vi "Main.vi"(8 "error in":errorcluster, 11 "Main UI in":refnum<class "Main UI.lvclass">) -> (0 "error out":errorcluster, 3 "Main UI out":refnum<class "Main UI.lvclass">)   [LabVIEW 2019, in "Main UI.lvclass"]
doc: "The <b>Queued Message Handler</b> of the Worker that owns this VI."
uses:
  Main UI.lvclass
  C:/Program Files (x86)/National Instruments/LabVIEW 2019/vi.lib/addons/_Workers/Library/Classes/Worker/Worker.lvclass
  Initialization Data.ctl
  Response Cases.ctl
  <vilib>/addons/_Workers/Library/Case Label.ctl
  Main UI.lvclass/Main UI.ctl
  rql_Start Motor.ctl
  <vilib>/addons/_Workers/Library/Classes/Message Queue/Message Queue.lvclass
  <vilib>/addons/_Workers/Library/Workers.lvlib
panel:
  in  "Start Motor":bool
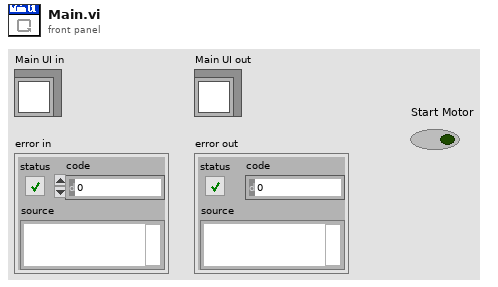
[diagram p1: front panel]
types:
  T1 = typedef "Main UI.lvclass/Initialization Data.ctl" = cluster{"Response Cases":T2}
  T2 = typedef "Main UI.lvclass/Response Cases.ctl" = cluster{"Placeholder - Can be deleted":string, "Start Motor":T3}
  T3 = typedef "Workers.lvlib/Case Label.ctl" = string
  T4 = typedef "Main UI.lvclass/rql_Start Motor.ctl" = cluster{"String":string}
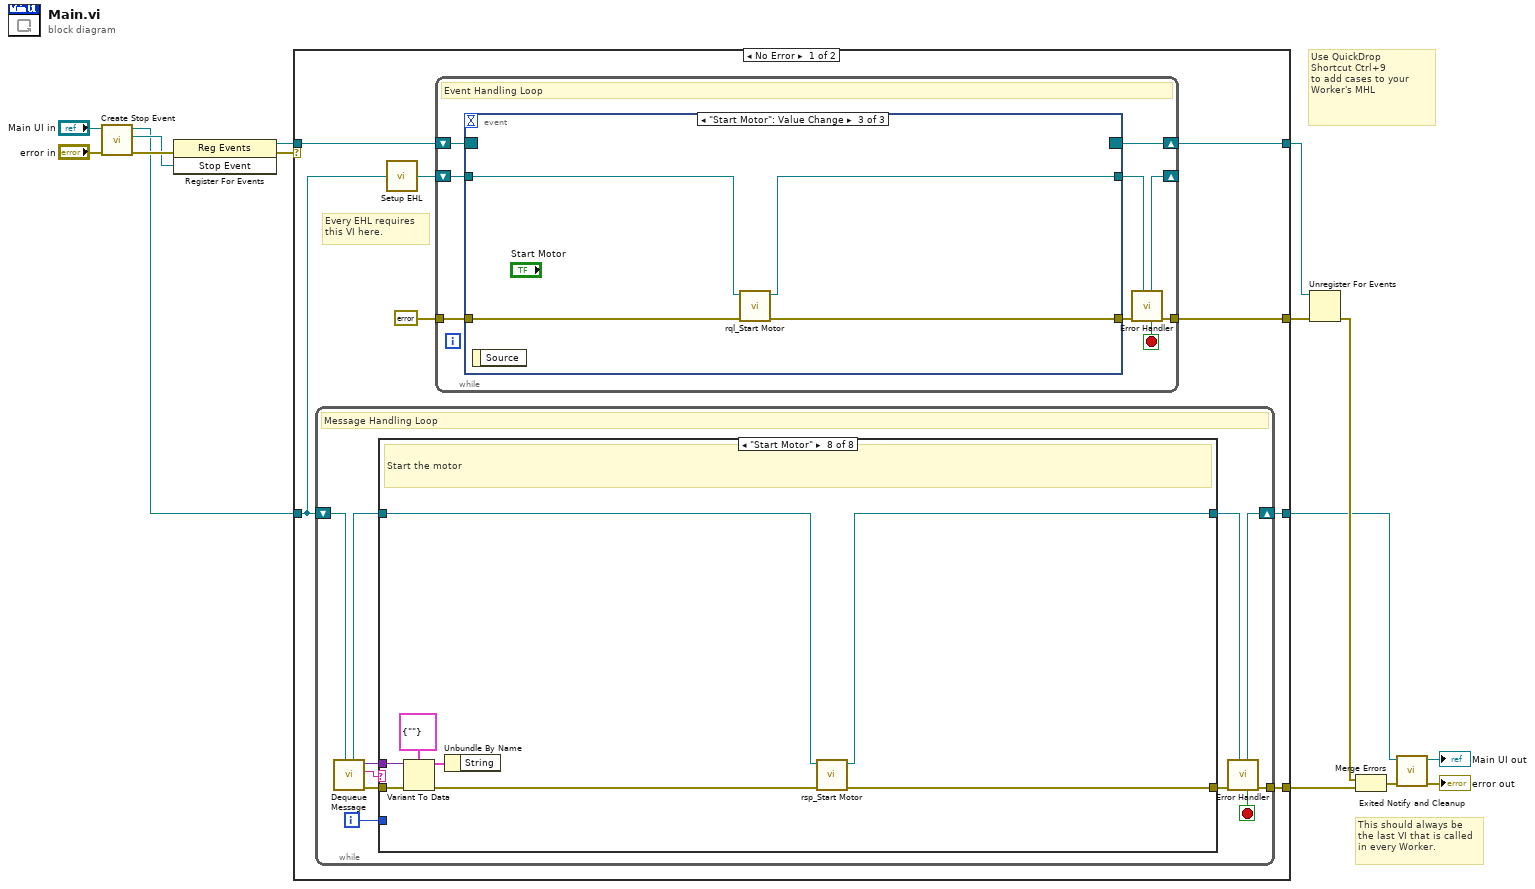
[diagram p0: block diagram]
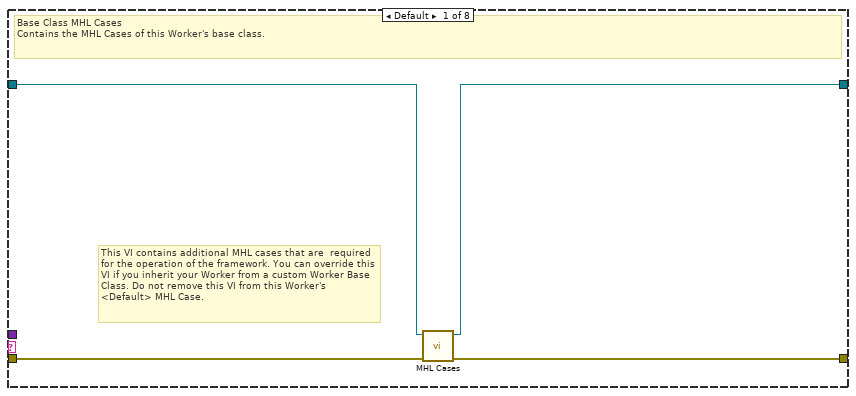
[diagram p2: hidden frame]
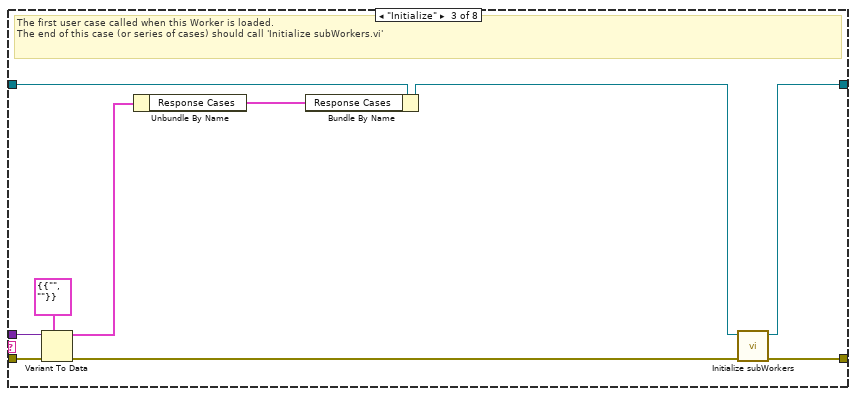
[diagram p4: hidden frame]
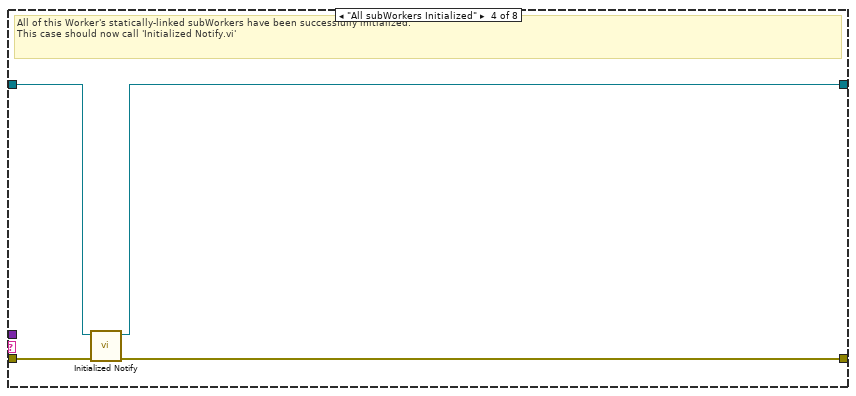
[diagram p5: hidden frame]
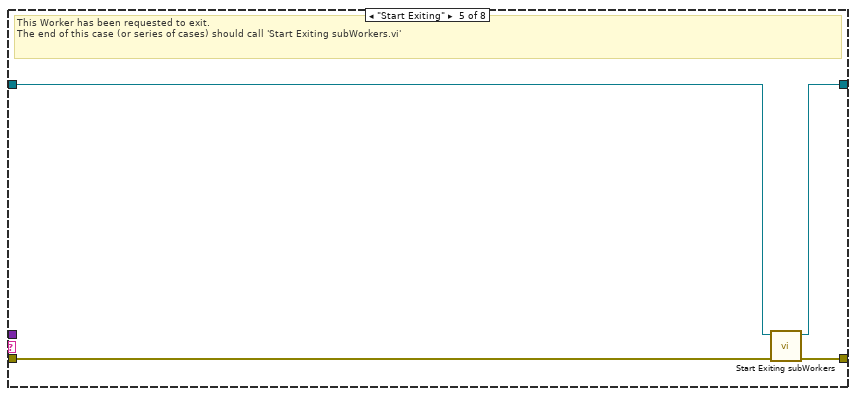
[diagram p6: hidden frame]
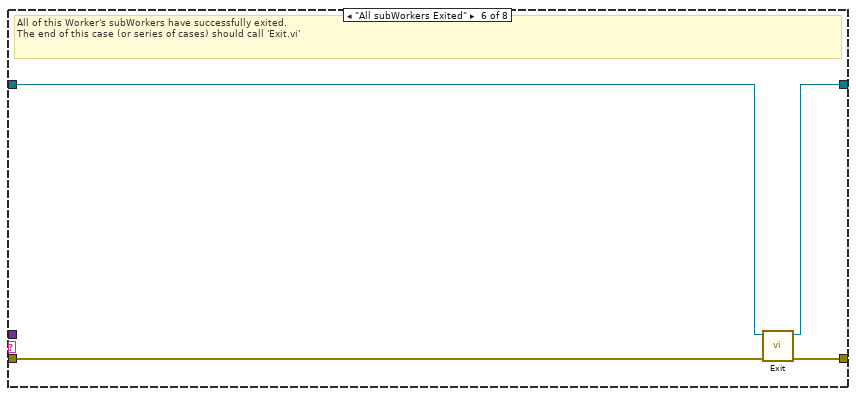
[diagram p7: hidden frame]
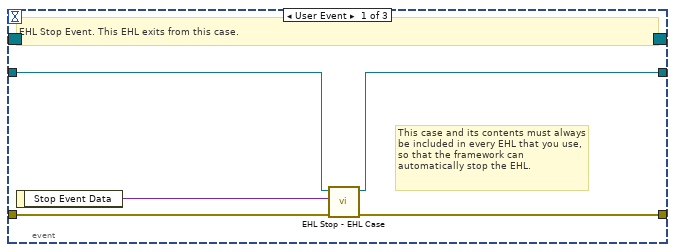
[diagram p9: hidden frame]
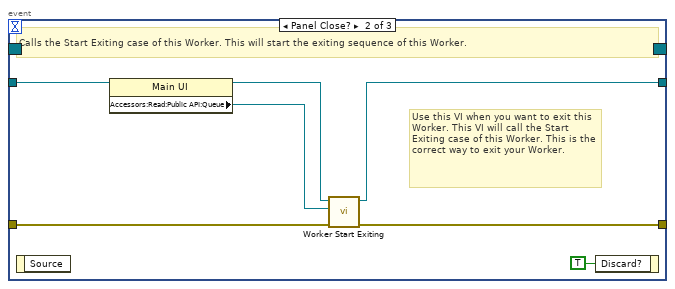
[diagram p10: hidden frame]
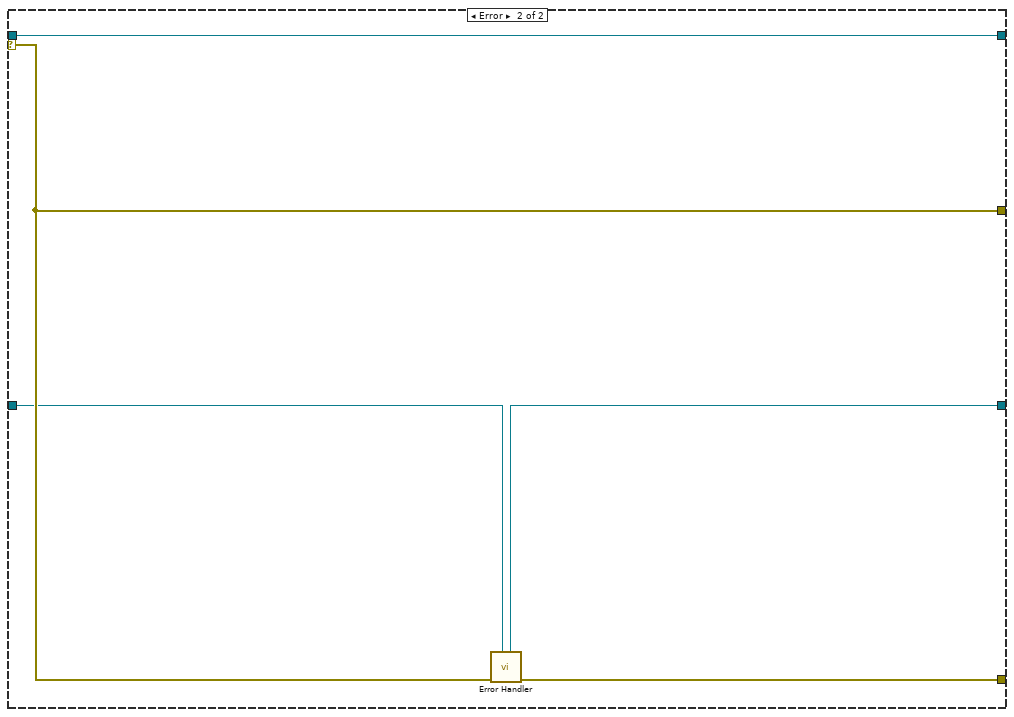
[diagram p11: hidden frame]
diagram:
  # "Use QuickDrop\nShortcut Ctrl+9\nto add cases to your\nWorker's MHL"
  # "This should always be the last VI that is called in every Worker."
  n1 = call-dynamic "Create Stop Event.vi"("error in"="error in", "Worker"="Main UI in") -> ("error out"=w10:errorcluster, "Stop Event"=w7:refnum<user-event>, "Worker out"=w4:refnum<class "Main UI.lvclass">)  [unwired: 7 in]
  n2 = register-events(error in=w10, w7) -> (reference out=w9:refnum<event-registration>, error out=w1:errorcluster)  [unwired: 1 in]
  n3 = case shown="No Error" w1 {
    tunnel: w4 -> [w18 w99]
    tunnel: [w16 w100] -> w8
    tunnel: w9 -> [w23 w101]
    tunnel: [w20 w102] -> w14
    tunnel: [w22 w101] -> w13
    tunnel: [w17 w98] -> w11
    selector: w1 -> [_ w102]
    frame No Error {
      # "Every EHL requires\nthis VI here."
      n4 = while {
        shift-right: [w32] -> w17
        shift-left: w18 -> [w34]
        tunnel: [w33] -> w16
        i -> [w25]
        stop <- w26 stop-if-true
        # "Message Handling Loop"
        n5 = call-dynamic "Dequeue Message.vi"("Worker"=w34) -> ("error out"=w31:errorcluster, "Case out"=w27:string, "Data out"=w24:variant, "Worker out"=w29:refnum<class "Main UI.lvclass">)  [unwired: 6 in, 1 out]
        n6 = case "Worker MHL Case Structure (DO NOT CHANGE LABEL NAME)" shown="\"Start Motor\"" w27 {
          tunnel: w31 -> [w38 w39 w48 w52 w55 w62 w64 w72]
          tunnel: [w37 w39 w50 w51 w58 w61 w64 w67] -> w30
          tunnel: w29 -> [w36 w40 w47 w54 w56 w60 w63 w66]
          tunnel: [w35 w40 w49 w53 w57 w59 w63 w65] -> w28
          tunnel: w25 -> [_ _ _ _ _ _ _ _]
          tunnel: w24 -> [_ _ w45 _ _ _ _ w70]
          frame Default {
            # "This VI contains additional MHL cases that are  required for the operation of the framework. You can override this VI if you inherit your Worker from a custom Worker Base Class. Do not remove this VI from this Worker's <Default> MHL Case."
            # "Base Class MHL Cases\nContains the MHL Cases of this Worker's base class."
            n7 = call-dynamic "MHL Cases.vi"("error in"=w38, "Worker in"=w36) -> ("error out"=w37:errorcluster, "Worker out"=w35:refnum<class "Main UI.lvclass">)  [unwired: 8 in]
          }
          frame "------------ FRAMEWORK CASES -----------" {
            # "Start of Workers Framework Cases"
          }
          frame "Initialize" {
            # "The first user case called when this Worker is loaded.\nThe end of this case (or series of cases) should call 'Initialize subWorkers.vi'"
            n8 = Variant To Data(error in=w48, type=T1 {"Response Cases"={"Placeholder - Can be deleted"="", "Start Motor"=""}} ("Initialization Data"), Variant=w45) -> (data=w43:T1, error out=w46:errorcluster)
            n9 = Unbundle By Name(w43) -> ("Response Cases"=w42:T2)
            n10 = Bundle By Name(cluster=w47, "Response Cases"=w42) -> (w44:refnum<class "Main UI.lvclass">)
            n11 = call-dynamic "Initialize subWorkers.vi"("error in"=w46, "Worker"=w44) -> ("error out"=w50:errorcluster, "dup Worker out"=w49:refnum<class "Main UI.lvclass">)  [unwired: 8 in]
          }
          frame "All subWorkers Initialized" {
            # "All of this Worker's statically-linked subWorkers have been successfully initialized.\nThis case should now call 'Initialized Notify.vi'"
            n12 = call-dynamic "Initialized Notify.vi"("error in"=w52, "Worker"=w54) -> ("error out"=w51:errorcluster, "dup Worker out"=w53:refnum<class "Main UI.lvclass">)  [unwired: 8 in]
          }
          frame "Start Exiting" {
            # "This Worker has been requested to exit. \nThe end of this case (or series of cases) should call 'Start Exiting subWorkers.vi'"
            n13 = call-dynamic "Start Exiting subWorkers.vi"("error_in"=w55, "Worker"=w56) -> ("error out"=w58:errorcluster, "dup Worker out"=w57:refnum<class "Main UI.lvclass">)  [unwired: 8 in]
          }
          frame "All subWorkers Exited" {
            # "All of this Worker's subWorkers have successfully exited. \nThe end of this case (or series of cases) should call 'Exit.vi'"
            n14 = call-dynamic "Exit.vi"("error_in"=w62, "Worker"=w60) -> ("error out"=w61:errorcluster, "dup Worker out"=w59:refnum<class "Main UI.lvclass">)  [unwired: 8 in]
          }
          frame "------------- LOCAL API CASES -------------" {
            # "Start of Workers Local API Cases"
          }
          frame "Start Motor" {
            # "Start the motor"
            n15 = Variant To Data(error in=w72, type=T4 {"String"=""} ("Data"), Variant=w70) -> (data=w69:T4, error out=w68:errorcluster)
            n16 = Unbundle By Name(w69) -> ()  [unwired: 1 out]
            n17 = call "rsp_Start Motor.vi"("error in"=w68, "Main UI in"=w66) -> ("error out"=w67:errorcluster, "dup Main UI out"=w65:refnum<class "Main UI.lvclass">)  [unwired: 8 in]
          }
        }
        n18 = call-dynamic "Error Handler.vi"("Worker"=w28, "error_in"=w30) -> ("error out"=w33:errorcluster, "Stop Loop"=w26:bool, "Worker out"=w32:refnum<class "Main UI.lvclass">)  [unwired: 7 in]
      }
      n19 = call-dynamic "Setup EHL.vi"("Worker"=w18) -> ("Worker out"=w19:refnum<class "Main UI.lvclass">)  [unwired: 14 in]
      n20 = while "Event Handling Loop" {
        shift-right: [w81] -> w22
        shift-left: w23 -> [w80]
        tunnel: [w76] -> w20
        tunnel: errorcluster {"status"=FALSE, "code"=0, "source"=""} ("error constant") -> [w78]
        shift-right: [w74] -> _
        shift-left: w19 -> [w79]
        stop <- w73 stop-if-true
        # "Event Handling Loop"
        n21 = event shown="[2] \"Start Motor\": Value Change" {
          selector: w80 -> [_ _ _]
          dyn-events: [_ _ _] -> w81
          timeout: _ -> [_ _ _]
          tunnel: [w85 w92 w96] -> w77
          tunnel: w78 -> [w86 w91 w97]
          tunnel: w79 -> [w84 w90 w95]
          tunnel: [w83 w89 w94] -> w75
          event User Event {
            # "This case and its contents must always be included in every EHL that you use, so that the framework can automatically stop the EHL."
            # "EHL Stop Event. This EHL exits from this case."
            n22 = event-data() -> ("Stop Event Data"=w82:variant)  [unwired: 1 in]
            n23 = call-dynamic "EHL Stop - EHL Case.vi"("error in"=w86, "Stop Event Data"=w82, "Worker"=w84) -> ("error out"=w85:errorcluster, "Worker out"=w83:refnum<class "Main UI.lvclass">)  [unwired: 7 in]
          }
          event Panel Close? {
            # "Use this VI when you want to exit this Worker. This VI will call the Start Exiting case of this Worker. This is the correct way to exit your Worker."
            # "Calls the Start Exiting case of this Worker. This will start the exiting sequence of this Worker."
            n24 = event-data() -> ()  [unwired: 1 in, 1 out]
            n25 = property class="Main UI"(reference=w90) -> (reference out=w88:refnum<class "Main UI.lvclass">, "Accessors:Read:Public API:Queue"=w87:refnum<class "Message Queue.lvclass">)  [unwired: 1 in, 1 out]
            n26 = call-dynamic "Worker Start Exiting.vi"("error_in"=w91, "Message Queue"=w87, "Worker"=w88) -> ("error out"=w92:errorcluster, "dup Worker out"=w89:refnum<class "Main UI.lvclass">)  [unwired: 7 in]
            n27 = event-data("Discard?"=TRUE) -> ()  [unwired: 1 in, 1 out]
          }
          event "Start Motor": Value Change {
            n28 = event-data() -> ()  [unwired: 1 in, 1 out]
            n29 = call "rql_Start Motor.vi"("error in"=w97, "Main UI in"=w95) -> ("error out"=w96:errorcluster, "dup Main UI out"=w94:refnum<class "Main UI.lvclass">)  [unwired: 8 in]
          }
        }
        n30 = call-dynamic "Error Handler.vi"("Worker"=w75, "error_in"=w77) -> ("error out"=w76:errorcluster, "Stop Loop"=w73:bool, "Worker out"=w74:refnum<class "Main UI.lvclass">)  [unwired: 7 in]
      }
    }
    frame Error {
      n31 = call-dynamic "Error Handler.vi"("Worker"=w99, "error_in"=w102) -> ("error out"=w100:errorcluster, "Worker out"=w98:refnum<class "Main UI.lvclass">)  [unwired: 7 in, 1 out]
    }
  }
  n32 = Unregister For Events(event registration refnum=w13, error in=w14) -> (error out=w15:errorcluster)
  n33 = Merge Errors(w15, w8) -> (w12:errorcluster)
  n34 = call-dynamic "Exited Notify and Cleanup.vi"("error_in"=w12, "Worker"=w11) -> ("error out"=→"error out":errorcluster, "dup Worker out"=→"Main UI out":refnum<class "Main UI.lvclass">)  [unwired: 8 in]
